vi "PE Get Library Version.vi"(8 "error in (no error)":errorcluster) -> (0 "error out":errorcluster, 3 "function return":i32)   [LabVIEW 2015, in "PE_Filter_SDK.lvlib"]
doc: "PEFILTERSDK_API int PE_GetLibraryVersion(void);"
uses:
  PE_Filter_SDK.lvlib
  Documents/test/SDK 1.2.4 Installer/SDK 1.2.4 Installer/win64/PE_Filter_SDK.dll
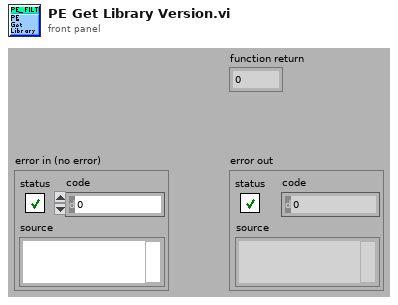
[diagram p1: front panel]
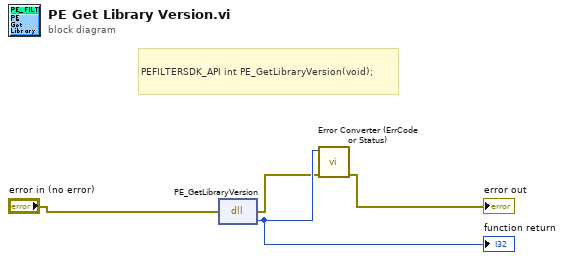
[diagram p0: block diagram]
diagram:
  # "PEFILTERSDK_API int PE_GetLibraryVersion(void);"
  n1 = dll-call lib="C:/Users/localAdmin/Documents/test/SDK 1.2.4 Installer/SDK 1.2.4 Installer/win64/PE_Filter_SDK.*" fn="PE_GetLibraryVersion"(error in="error in (no error)") -> (error out=w2:errorcluster, w4:i32)  [unwired: 2 in, 1 out]
  "function return" <- w4
  n2 = call "Error Converter (ErrCode or Status).vi"("error in (no error)"=w2, "error code"=w4) -> ("error out"=→"error out":errorcluster)  [unwired: 9 in]
